vi "Mode Page.vi"(8 "Error in":errorcluster, 11 "INL DNL Test In":refnum<class "INL DNL Test.lvclass">) -> (0 "Error out":errorcluster, 3 "INL DNL Test Out":refnum<class "INL DNL Test.lvclass">)   [LabVIEW 2020, in "INL DNL Test.lvclass"]
doc: "Mode page to select the device mode and enter the device values."
uses:
  INL DNL Test.lvclass
  D:/INL DNL Test/Class/Test/Parent/Test.lvclass
  Parent/Typedef/User Event Controls.ctl
  Parent/Typedef/Queue Driver Controls.ctl
  Device/Parent/Device.lvclass
  Parent/Test.lvclass
panel:
  in  "Error Rate (in %)":dbl=25.0 min=0.0 max=100.0
  in  "Voltage (V)":dbl=8.0 min=0.0
  in  "Resolution":dbl=3.0 min=1.0 max=6.0
  in  "DAC":bool caption="Digital to Analog converter"
  in  "ADC":bool caption="Analog to digital converter"
  # "Note:\n1. Choose the mode to calculate INL and DNl result\n2. Enter the parameter values for the calculation"
  # "Choose the mode"
  # "Enter parameters"
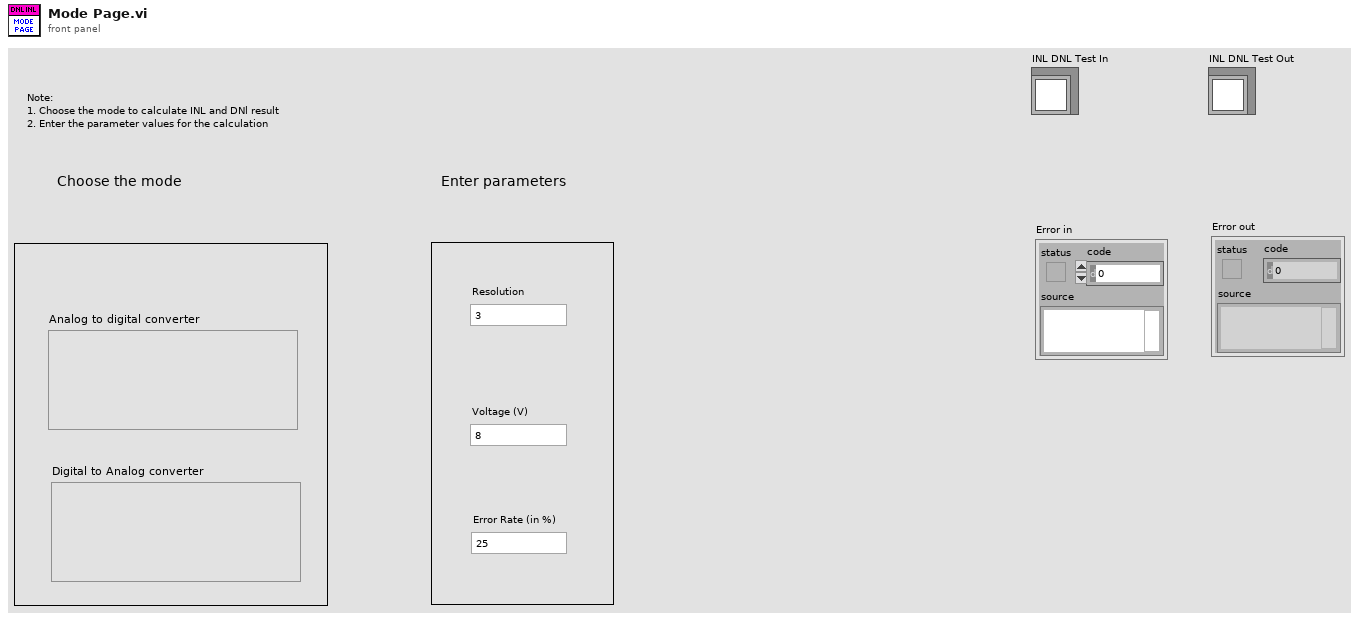
[diagram p1: front panel]
types:
  T1 = typedef "Test.lvclass/Queue Driver Controls.ctl" = enum16{"Create Queue", "Enqueue", "Dequeue", "Enstack", "Flush Queue", "Release Queue"}
  T2 = typedef "Test.lvclass/User Event Controls.ctl" = enum16{"Create", "Generate", "Run Test", "Get Ref", "Destroy"}
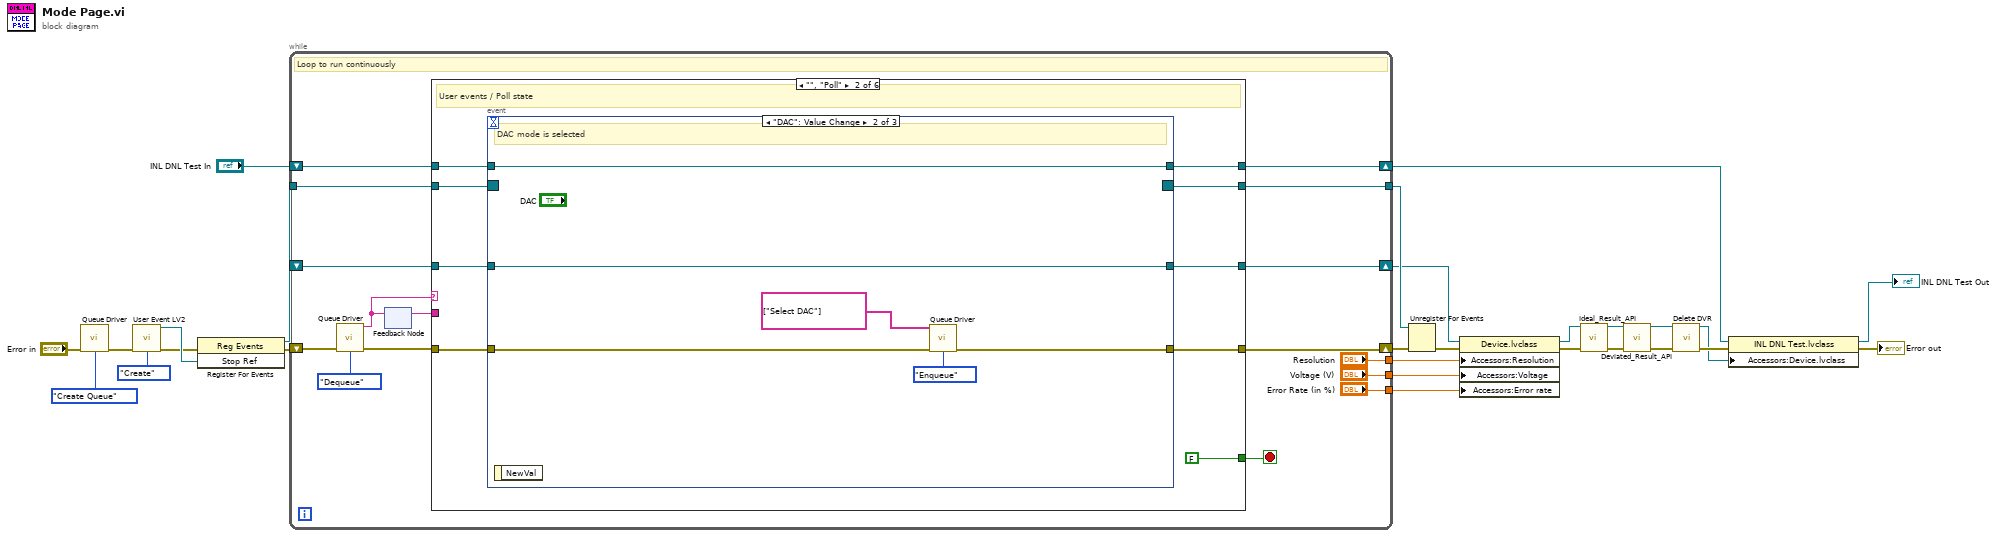
[diagram p0: block diagram]
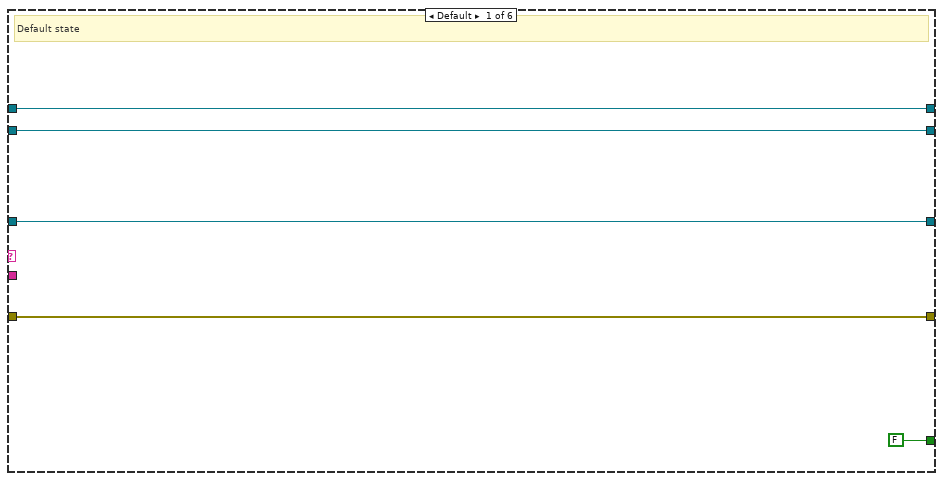
[diagram p2: hidden frame]
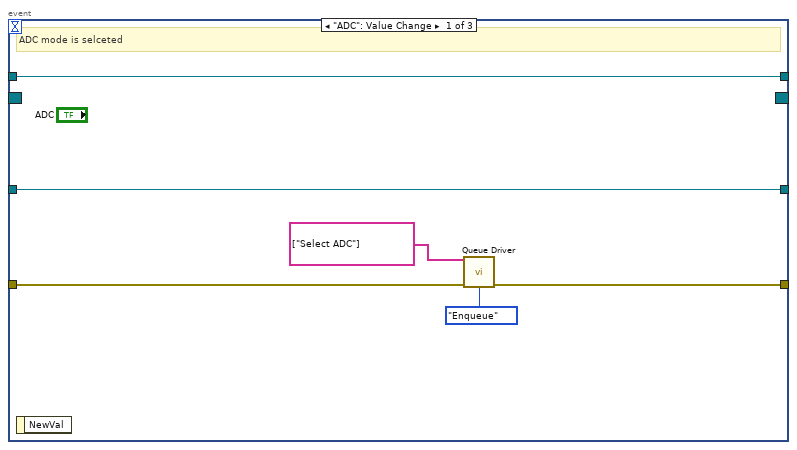
[diagram p3: hidden frame]
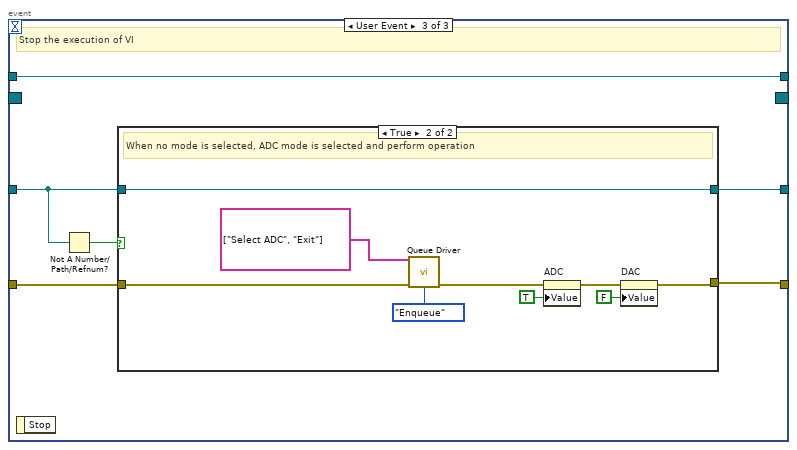
[diagram p4: hidden frame]
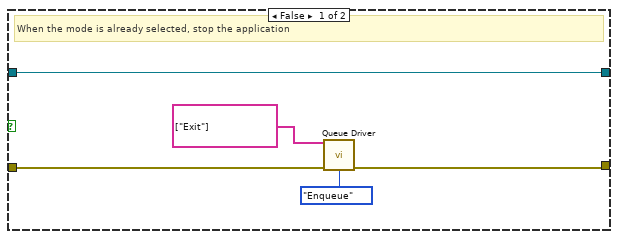
[diagram p5: hidden frame]
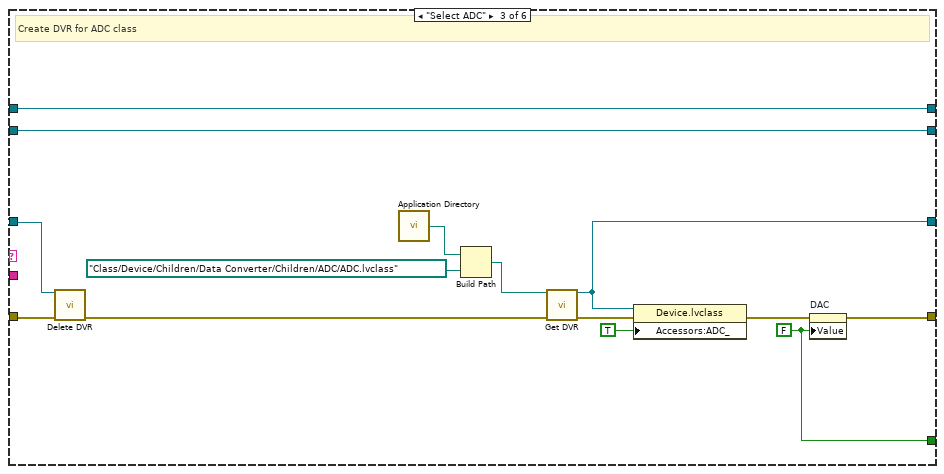
[diagram p6: hidden frame]
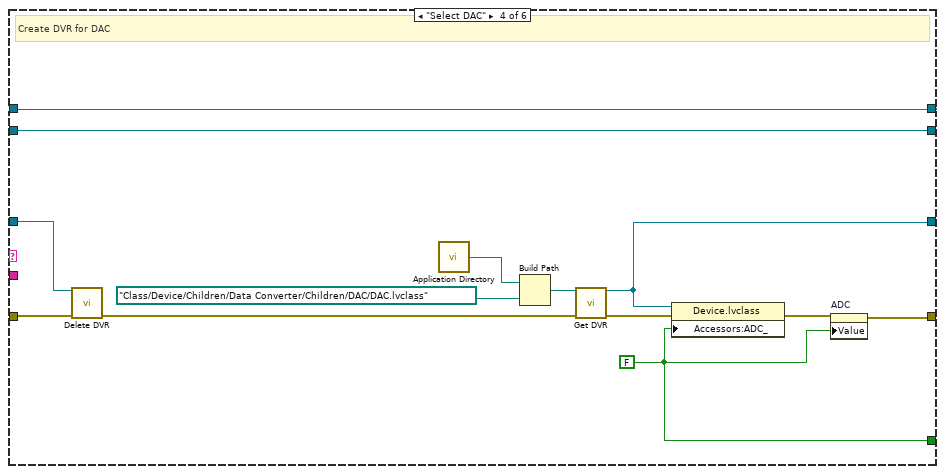
[diagram p7: hidden frame]
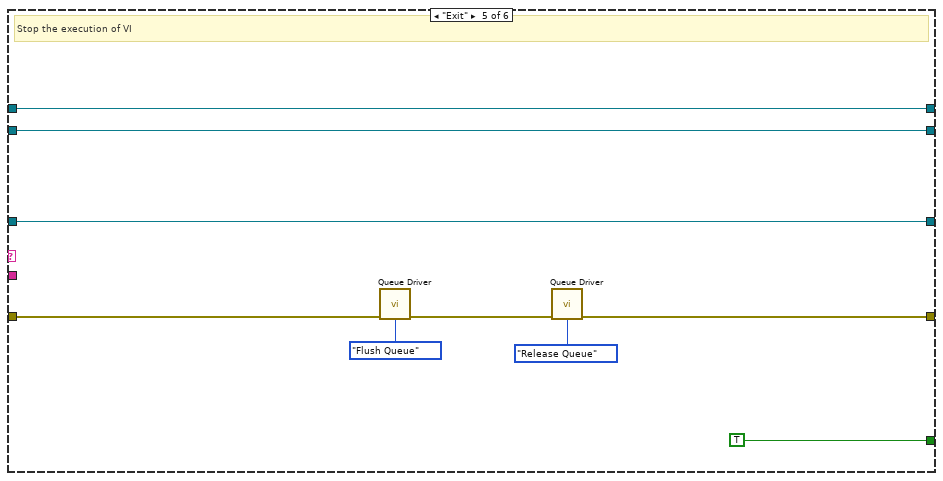
[diagram p8: hidden frame]
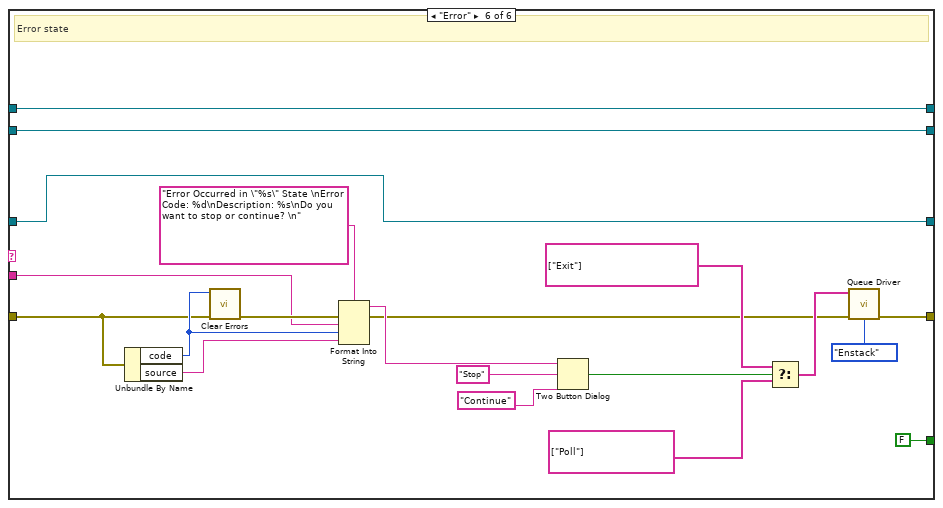
[diagram p9: hidden frame]
diagram:
  n1 = call "Queue Driver.vi"("Error in"="Error in", "Queue Controls"=Queue_Driver_Controls."Create Queue") -> ("Error out"=w4:errorcluster)  [unwired: 12 in, 1 out]
  n2 = call "User Event LV2.vi"("Error In"=w4, "User event controls"=User_Event_Controls."Create") -> ("Stop Ref"=w8:refnum<user-event>, "Error Out"=w7:errorcluster)  [unwired: 11 in, 1 out]
  n3 = register-events(error in=w7, w8) -> (reference out=w27:refnum<event-registration>, error out=w26:errorcluster)  [unwired: 1 in]
  n4 = while {
    tunnel: w27 -> [w43]
    shift-right: [w41] -> w18
    shift-left: "INL DNL Test In" -> [w42]
    shift-right: [w40] -> w25
    shift-left: w26 -> [w30]
    tunnel: [w39] -> w23
    shift-right: [w38] -> w22
    shift-left: _ -> [w37]
    tunnel: ["Resolution"] -> w11
    tunnel: ["Error Rate (in %)"] -> w10
    tunnel: ["Voltage (V)"] -> w9
    stop <- w36 stop-if-true
    # "Loop to run continuously"
    n5 = call "Queue Driver.vi"("Error in"=w30, "Queue Controls"=Queue_Driver_Controls."Dequeue") -> ("Dequeue Element"=w31:string, "Error out"=w29:errorcluster)  [unwired: 12 in]
    n6 = feedback-in #1(w31) -> ()
    n7 = feedback #1() -> (w32:string)  [unwired: 1 in]
    n8 = case shown="\"\", \"Poll\"" w31 {
      tunnel: w43 -> [w45 w57 w93 w108 w124 w132]
      tunnel: w29 -> [w46 w56 w98 w113 w121 w135]
      tunnel: w42 -> [w48 w55 w94 w109 w125 w131]
      tunnel: [w48 w54 w94 w109 w125 w131] -> w41
      tunnel: [w46 w53 w95 w110 w118 w127] -> w40
      tunnel: [w45 w52 w93 w108 w124 w132] -> w39
      tunnel: [w47 w51 w96 w111 w123 w133] -> w38
      tunnel: w37 -> [w47 w50 w97 w112 w123 w133]
      tunnel: [FALSE FALSE w92 w107 TRUE FALSE ("ADC_")] -> w36
      tunnel: w32 -> [_ _ _ _ _ w134]
      frame Default {
        # "Default state"
      }
      frame "", "Poll" {
        # "User events / Poll state"
        n9 = event shown="[1] \"DAC\": Value Change" {
          selector: w57 -> [_ _ _]
          dyn-events: [_ _ _] -> w52
          timeout: _ -> [_ _ _]
          tunnel: w56 -> [w61 w67 w75]
          tunnel: w55 -> [w63 w69 w74]
          tunnel: [w63 w69 w74] -> w54
          tunnel: [w60 w66 w73] -> w53
          tunnel: [w62 w68 w72] -> w51
          tunnel: w50 -> [w62 w68 w70]
          event "ADC": Value Change {
            # "ADC mode is selceted"
            n10 = event-data() -> ()  [unwired: 1 in, 1 out]
            n11 = call "Queue Driver.vi"("States"=string[] ["Select ADC"], "Error in"=w61, "Queue Controls"=Queue_Driver_Controls."Enqueue") -> ("Error out"=w60:errorcluster)  [unwired: 11 in, 1 out]
          }
          event "DAC": Value Change {
            # "DAC mode is selected"
            n12 = event-data() -> ()  [unwired: 1 in, 1 out]
            n13 = call "Queue Driver.vi"("States"=string[] ["Select DAC"], "Error in"=w67, "Queue Controls"=Queue_Driver_Controls."Enqueue") -> ("Error out"=w66:errorcluster)  [unwired: 11 in, 1 out]
          }
          event User Event {
            # "Stop the execution of VI"
            n14 = event-data() -> ()  [unwired: 1 in, 1 out]
            n15 = Not A Number/Path/Refnum?(number/path/refnum=w70) -> (NaN/Path/Refnum?=w71:bool)
            n16 = case shown="True" w71 {
              tunnel: w75 -> [w79 w89]
              tunnel: [w76 w85] -> w73
              tunnel: w70 -> [w80 w88]
              tunnel: [w80 w88] -> w72
              frame False {
                # "When the mode is already selected, stop the application"
                n17 = call "Queue Driver.vi"("States"=string[] ["Exit"], "Error in"=w79, "Queue Controls"=Queue_Driver_Controls."Enqueue") -> ("Error out"=w76:errorcluster)  [unwired: 11 in, 1 out]
              }
              frame True {
                # "When no mode is selected, ADC mode is selected and perform operation"
                n18 = call "Queue Driver.vi"("States"=string[] ["Select ADC", "Exit"], "Error in"=w89, "Queue Controls"=Queue_Driver_Controls."Enqueue") -> ("Error out"=w83:errorcluster)  [unwired: 11 in, 1 out]
                n19 = property on="ADC" class="Bool (strict)"(error in=w83, "Value"=TRUE ("ADC")) -> (error out=w87:errorcluster)  [unwired: 1 in, 1 out]
                n20 = property on="DAC" class="Bool (strict)"(error in=w87, "Value"=FALSE ("DAC")) -> (error out=w85:errorcluster)  [unwired: 1 in, 1 out]
              }
            }
          }
        }
      }
      frame "Select ADC" {
        w92 = FALSE ("Digital to Analog converter")
        # "Create DVR for ADC class"
        n21 = call "Delete DVR.vi"("Device DVR"=w97, "Error in"=w98) -> ("Error out"=w101:errorcluster)  [unwired: 12 in, 1 out]
        n22 = call <vilib>:"Application Directory.vi"() -> ("Application Directory"=w90:path)
        n23 = Build Path(base path=w90, name or relative path=path "Class/Device/Children/Data Converter/Children/ADC/ADC.lvclass") -> (appended path=w102:path)
        n24 = call "Get DVR.vi"("Class Path"=w102, "Error in"=w101) -> ("Device DVR"=w96:refnum<data-value>, "Error out"=w103:errorcluster)  [unwired: 12 in]
        n25 = property class="Device.lvclass"(reference=w96, error in=w103, "Accessors:ADC_"=TRUE ("ADC_")) -> (error out=w100:errorcluster)  [unwired: 1 out]
        n26 = property on="DAC" class="Bool (strict)"(error in=w100, "Value"=w92) -> (error out=w95:errorcluster)  [unwired: 1 in, 1 out]
      }
      frame "Select DAC" {
        w107 = FALSE ("ADC_")
        # "Create DVR for DAC"
        n27 = call "Delete DVR.vi"("Device DVR"=w112, "Error in"=w113) -> ("Error out"=w104:errorcluster)  [unwired: 12 in, 1 out]
        n28 = call <vilib>:"Application Directory.vi"() -> ("Application Directory"=w105:path)
        n29 = Build Path(base path=w105, name or relative path=path "Class/Device/Children/Data Converter/Children/DAC/DAC.lvclass") -> (appended path=w115:path)
        n30 = call "Get DVR.vi"("Class Path"=w115, "Error in"=w104) -> ("Device DVR"=w111:refnum<data-value>, "Error out"=w116:errorcluster)  [unwired: 12 in]
        n31 = property class="Device.lvclass"(reference=w111, error in=w116, "Accessors:ADC_"=w107) -> (error out=w114:errorcluster)  [unwired: 1 out]
        n32 = property on="ADC" class="Bool (strict)"(error in=w114, "Value"=w107) -> (error out=w110:errorcluster)  [unwired: 1 in, 1 out]
      }
      frame "Exit" {
        # "Stop the execution of VI"
        n33 = call "Queue Driver.vi"("Error in"=w121, "Queue Controls"=Queue_Driver_Controls."Flush Queue") -> ("Error out"=w120:errorcluster)  [unwired: 12 in, 1 out]
        n34 = call "Queue Driver.vi"("Error in"=w120, "Queue Controls"=Queue_Driver_Controls."Release Queue") -> ("Error out"=w118:errorcluster)  [unwired: 12 in, 1 out]
      }
      frame "Error" {
        # "Error state"
        n35 = Unbundle By Name(w135) -> ("code"=w143:i32, "source"=w142:string)
        n36 = call <vilib>:"Clear Errors.vi"("error in (no error)"=w135, "specific error code to clear (0: all)"=w143) -> ("error out"=w145:errorcluster)  [unwired: 4 in, 1 out]
        n37 = Format Into String(format string="Error Occurred in \"%s\" State \nError Code: %d\nDescription: %s\nDo you want to stop or continue? \n", error in=w145, w134, w143, w142) -> (resulting string=w141:string, error out=w128:errorcluster)  [unwired: 1 in]
        n38 = Two Button Dialog(message=w141, 1:"Continue" ("F button name (\"Cancel\")"), 2:"Stop" ("T button name (\"OK\")")) -> (T button?=w138:bool)
        n39 = Select(t=string[] ["Exit"] ("States"), s=w138, f=string[] ["Poll"] ("States")) -> (s? t:f=w129:string[])
        n40 = call "Queue Driver.vi"("States"=w129, "Error in"=w128, "Queue Controls"=Queue_Driver_Controls."Enstack") -> ("Error out"=w127:errorcluster)  [unwired: 11 in, 1 out]
      }
    }
  }
  n41 = Unregister For Events(event registration refnum=w23, error in=w25) -> (error out=w24:errorcluster)
  n42 = property class="Device.lvclass"(reference=w22, error in=w24, "Accessors:Resolution"=w11, "Accessors:Voltage"=w9, "Accessors:Error rate"=w10) -> (reference out=w20:refnum<data-value>, error out=w21:errorcluster)
  n43 = call "Ideal_Result_API.vi"("Device DVR"=w20, "Error in"=w21) -> ("Device DVR"=w14:refnum<data-value>, "Error Out"=w15:errorcluster)  [unwired: 12 in]
  n44 = call "Deviated_Result_API.vi"("Device DVR In"=w14, "Error in"=w15) -> ("Device DVR Out"=w12:refnum<data-value>, "Error Out"=w13:errorcluster)  [unwired: 12 in]
  n45 = call "Delete DVR.vi"("Device DVR"=w12, "Error in"=w13) -> ("Device Class Out"=w17:refnum<class "Device.lvclass">, "Error out"=w19:errorcluster)  [unwired: 12 in]
  n46 = property class="INL DNL Test.lvclass"(reference=w18, error in=w19, "Accessors:Device.lvclass"=w17) -> (reference out=→"INL DNL Test Out":refnum<class "INL DNL Test.lvclass">, error out=→"Error out":errorcluster)
